vi "ATF-Display & Datalog.vi"() -> ()   [LabVIEW 2022 SP3]
uses:
  Source Code/Globals/SeCrTS-DD globals.vi
  0df20dd4-2c00-4f15-959c-8f534c1a7d29.vi
  97d5b880-568e-4530-a46e-1f8a36fc1bc1.vi
panel:
  out "log heath":bool
  out "Connected?":bool
  in  "IP ADDRESS":string="169.254.92.110"
  out "error out":errorcluster
  in  "error in":errorcluster
  # "DISPLAY & DATALOG V1.0"
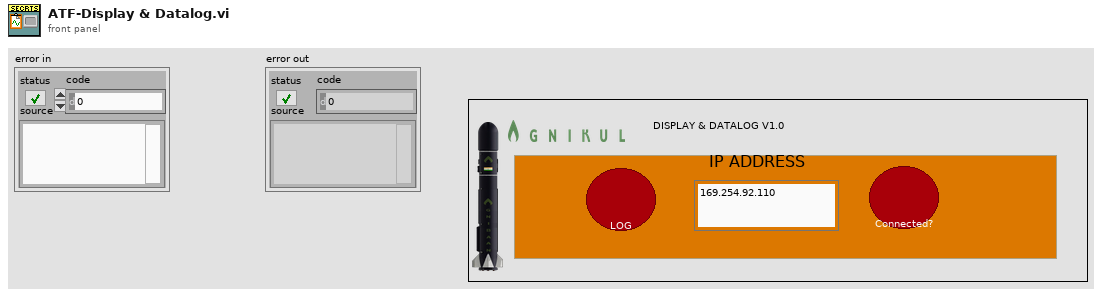
[diagram p1: front panel]
types:
  T1 = cluster{"AO config":cluster{"Channel_Name":string, "Channel_Number":string, "Default_Value":dbl, "Units":string}[], "AI config":cluster{"Channel_Name":string, "Channel_Number":string, "Pre_Scale_min":dbl, "Pre_Scale_max":dbl, "Sensor_min":dbl, "Sensor_max":dbl, "Units":string}[], "DI config":cluster{"Channel_Name":string, "Channel_Number":string, "Default_Value":bool, "DI invert?":bool}[], "DO config":cluster{"Channel_Name":string, "Channel_Number":string, "Default_Value":bool, "DO invert?":bool}[], "TC config":cluster{"Channel_Name":string, "Channel_Number":string, "Pre_Scale_min":dbl, "Pre_Scale_max":dbl, "units":i32, " type":i32}[], "ACC config":cluster{"Channel_Name":string, "Channel_Number":string, "Pre_Scale_min":dbl, "Pre_Scale_max":dbl, "Terminal configuration":i32, "Sensitivity":dbl, "Sensitivity units":i32}[], "SG config":cluster{"Channel_Name":string, "Channel_Number":string, "Pre_Scale_min":dbl, "Pre_Scale_max":dbl}[], "Strain Gauge Settings":cluster{"poisson ratio":dbl, "nominal gage resistance":dbl, "gage factor":dbl}, "Bridge Settings":cluster{"voltage excitation value":dbl, "voltage excitation source":i32, "initial bridge voltage":dbl, "lead wire resistance":dbl, "strain configuration":i32}, "Sample Rate":cluster{"AI Sample Rate":dbl[], "AO Sample Rate":dbl[], "DI Sample Rate":dbl[], "TC Sample Rate":dbl[], "DO Sample Rate":dbl[], "SG Sample Rate":dbl[], "ACC Sample Rate":dbl[]}}
  T2 = cluster{"analog names":cluster{"AI_C_Data":string[], "AI_V_Data":string[], "AO_Data":string[], "DO_Data":string[], "ACC_Data":string[], "TC Data":string[], "Drive_A_C":string[], "Drive_A_D":string[], "Drive_L_C":string[], "Drive_L_D":string[]}, "Di names":string[]}
  T3 = cluster{"Channel names":cluster{"AI_C_Data P":string[], "AI_V_Data P":string[], "AO_Data P":string[], "DO_Data P":string[], "ACC_Data P":string[], "TC Data P":string[], "Drive_A_C":string[], "Drive_A_D":string[], "AI_C_Data S":string[], "DO_Data S":string[]}, "DI Names":cluster{"Di P":string[], "Di S":string[]}}
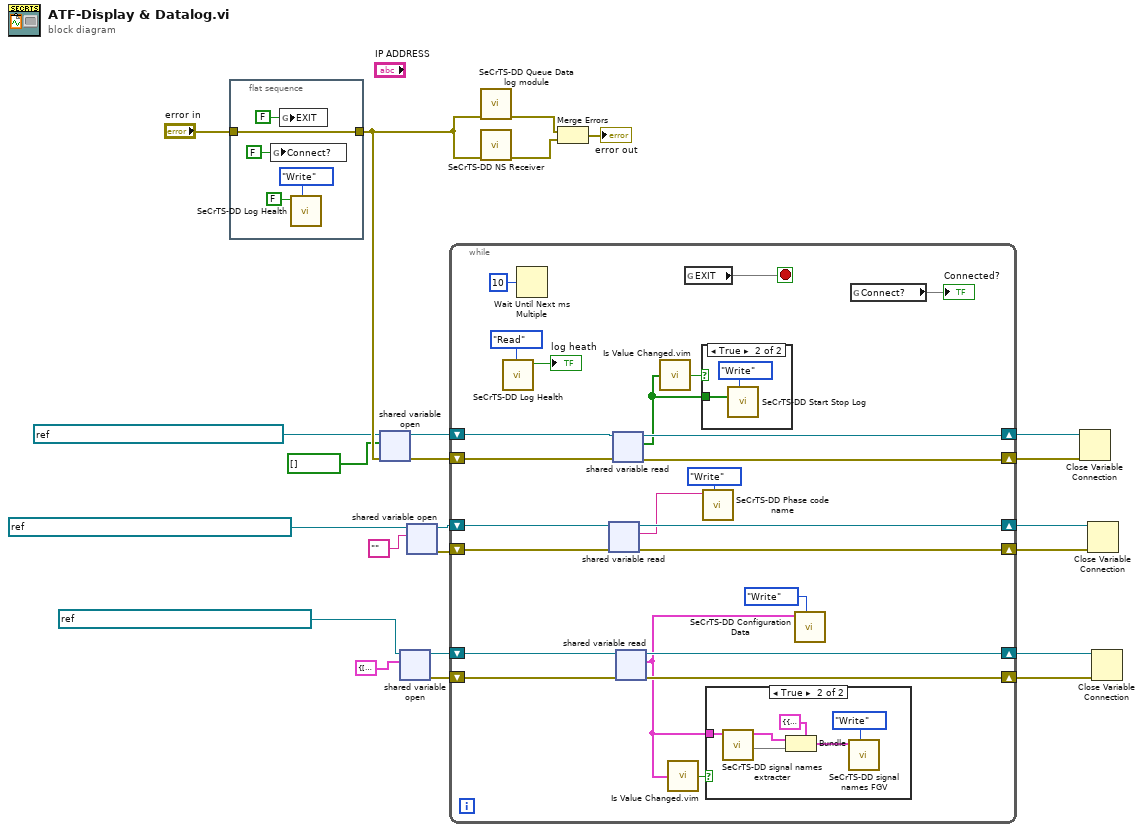
[diagram p0: block diagram]
diagram:
  n1 = flat-sequence {
    tunnel: "error in" -> [w27]
    tunnel: [w27] -> w19
    frame #0 {
      n2 = global write "SeCrTS-DD globals.vi" "Connect?"(FALSE ("Connect?")) -> ()
      n3 = global write "SeCrTS-DD globals.vi" "EXIT"(FALSE ("EXIT")) -> ()
      n4 = call "SeCrTS-DD Log Health.vi"("Enum"=enum16{"Read", "Write"}."Write", "Log health"=FALSE) -> ()  [unwired: 8 in, 2 out]
    }
  }
  n5 = shared-variable-open(refnum<k21> "ni.var.psp://tto-pxie/Device/Start Stop log" ("shared variable refnum in"), w19, bool[] []) -> (w15:refnum<k21>, w14:errorcluster)  [unwired: 1 in]
  n6 = shared-variable-open(refnum<k21> "ni.var.psp://tto-pxie/Device/Configuration" ("shared variable refnum in"), T1 {"AO config"=[], "AI config"=[], "DI config"=[], "DO config"=[], "TC config"=[], "ACC config"=[], "SG config"=[], "Strain Gauge Settings"={"poisson ratio"=0.3, "nominal gage resistance"=120.0, "gage factor"=2.08}, "Bridge Settings"={"voltage excitation value"=3.3, "voltage excitation source"=10200, "initial bridge voltage"=0.0, "lead wire resistance"=1.7, "strain configuration"=10271}, "Sample Rate"={"AI Sample Rate"=[], "AO Sample Rate"=[], "DI Sample Rate"=[], "TC Sample Rate"=[], "DO Sample Rate"=[], "SG Sample Rate"=[], "ACC Sample Rate"=[]}} ("data")) -> (w6:refnum<k21>, w4:errorcluster)  [unwired: 2 in]
  n7 = shared-variable-open(refnum<k21> "ni.var.psp://tto-pxie/Device/Datalog phase code" ("shared variable refnum in"), "") -> (w10:refnum<k21>, w9:errorcluster)  [unwired: 2 in]
  n8 = while "Monitoring" {
    shift-right: [w47] -> w13
    shift-left: w15 -> [w48]
    shift-right: [w45] -> w12
    shift-left: w14 -> [w46]
    shift-right: [w42] -> w7
    shift-left: w10 -> [w44]
    shift-right: [w41] -> w8
    shift-left: w9 -> [w43]
    shift-right: [w33] -> w2
    shift-left: w6 -> [w36]
    shift-right: [w32] -> w1
    shift-left: w4 -> [w35]
    stop <- w29 stop-if-true
    (unwired) enum16{"Read", "Write"}."Read" ("Enum")
    n9 = call "SeCrTS-DD Log Health.vi"("Enum"=enum16{"Read", "Write"}."Read") -> ("Log health R"=→"log heath":bool)  [unwired: 9 in, 1 out]
    n10 = Wait Until Next ms Multiple(millisecond multiple=u32 10) -> ()  [unwired: 1 out]
    n11 = shared-variable-read(w44, w43) -> (w42:refnum<k21>, w41:errorcluster, w39:string)  [unwired: 1 out]
    n12 = shared-variable-read(w48, w46) -> (w47:refnum<k21>, w45:errorcluster, w37:bool[])  [unwired: 1 out]
    n13 = shared-variable-read(w36, w35) -> (w33:refnum<k21>, w32:errorcluster, w31:T1)  [unwired: 1 out]
    n14 = call "Is Value Changed.vim"("value"=w37) -> ("changed or first call?"=w38:bool)
    n15 = call "Is Value Changed.vim"("value"=w31) -> ("changed or first call?"=w30:bool)
    n16 = global read "SeCrTS-DD globals.vi" "EXIT"() -> (w29)
    n17 = case shown="True" w38 {
      tunnel: w37 -> [_ w59]
      frame False {
      }
      frame True {
        n18 = call "SeCrTS-DD Start Stop Log.vi"("Enum"=enum16{"Read", "Write"}."Write", "Start Stop log"=w59) -> ()  [unwired: 8 in, 2 out]
      }
    }
    n19 = call "SeCrTS-DD Phase code name.vi"("Enum"=enum16{"Read", "Write"}."Write", "Phase code W"=w39) -> ()  [unwired: 8 in, 2 out]
    n20 = case shown="True" w30 {
      tunnel: w31 -> [_ w58]
      frame False {
      }
      frame True {
        n21 = call "SeCrTS-DD signal names extracter.vi"("input cluster"=w58) -> (1:w55, "Signal names"=w56:T3)  [unwired: 9 in]
        n22 = Bundle(cluster=T2 {"analog names"={"AI_C_Data"=[], "AI_V_Data"=[], "AO_Data"=[], "DO_Data"=[], "ACC_Data"=[], "TC Data"=[], "Drive_A_C"=[], "Drive_A_D"=[], "Drive_L_C"=[], "Drive_L_D"=[]}, "Di names"=[]}, "analog names"=w56, "Di names"=w55) -> (w54:T2)
        n23 = call "SeCrTS-DD signal names FGV.vi"("Enum"=enum16{"Read", "Write"}."Write", "Signal names"=w54) -> ()  [unwired: 8 in, 2 out]
      }
    }
    n24 = call "SeCrTS-DD Configuration Data.vi"("Enum"=enum16{"Read", "Write"}."Write", "data"=w31) -> ()  [unwired: 8 in, 2 out]
    n25 = global read "SeCrTS-DD globals.vi" "Connect?"() -> (→"Connected?")
  }
  n26 = call "SeCrTS-DD Queue Data log module.vi"("error in"=w19) -> ("error out"=w23:errorcluster)  [unwired: 10 in]
  n27 = call "SeCrTS-DD NS Receiver.vi"("error in"=w19) -> ("error out"=w22:errorcluster)  [unwired: 10 in]
  n28 = Merge Errors(w23, w22) -> (→"error out":errorcluster)
  n29 = Close Variable Connection(8:w12, 11:w13) -> ()  [unwired: 1 out]
  n30 = Close Variable Connection(8:w8, 11:w7) -> ()  [unwired: 1 out]
  n31 = Close Variable Connection(8:w1, 11:w2) -> ()  [unwired: 1 out]
